vi "OHLayerGen.vi"(6 "Layer":u32=160, 8 "OHL2pow":dbl=150.0, 9 "OHL1pow":dbl=75.0, 10 "HatchPow":T5={"Power"=300.0, "Mark Speed"=400.0, "Jump Speed"=1000.0}, 11 "RectHatch":T6={"Width"=10.0, "Height"=10.0, "Angle"=45.0, "OffX"=0.1, "OffY"=0.1, "Spacing"=0.1} {"Spacing" format="%#_13g"; "OffY" format="%#_13g"; "OffX" format="%#_13g"; "Height" format="%#_13g"; "Width" format="%#_13g"}) -> (3 "PathSups":T1[](array[typedef]))   [LabVIEW 2014]
uses:
  TypeDefs/RectHatch.ctl
  TypeDefs/PowerSpeed.ctl
  TypeDefs/PathSupreme.ctl
  PSup2SCAN/Sub/VelocityProfile.ctl
  PSup2SCAN/Sub/PathCut.ctl
  PSup2SCAN/Sub/Segment.ctl
  PSup2SCAN/Sub/Point.ctl
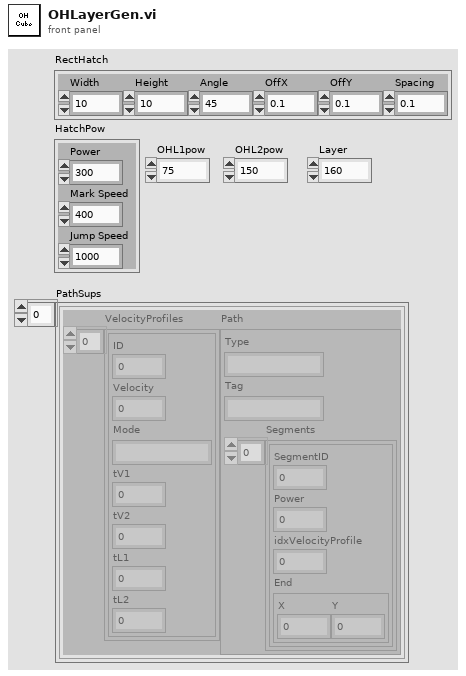
[diagram p1: front panel]
types:
  T1 = typedef "PathSupreme.ctl" = cluster{"VelocityProfiles":T2[], "Path":T3}
  T2 = typedef "VelocityProfile.ctl" = cluster{"ID":u32, "Velocity":dbl, "Mode":string, "tV1":u32, "tV2":u32, "tL1":u32, "tL2":u32}
  T3 = typedef "PathCut.ctl" = cluster{"Type":string, "Tag":string, "Segments":T4[]}
  T4 = typedef "Segment.ctl" = cluster{"SegmentID":u16, "Power":sgl, "idxVelocityProfile":u16, "End":cluster{"X":sgl, "Y":sgl}}
  T5 = typedef "PowerSpeed.ctl" = cluster{"Power":dbl, "Mark Speed":dbl, "Jump Speed":dbl}
  T6 = typedef "RectHatch.ctl" = cluster{"Width":dbl, "Height":dbl, "Angle":sgl, "OffX":dbl, "OffY":dbl, "Spacing":dbl}
  T7 = typedef "Point.ctl" = cluster{"X":dbl, "Y":dbl}
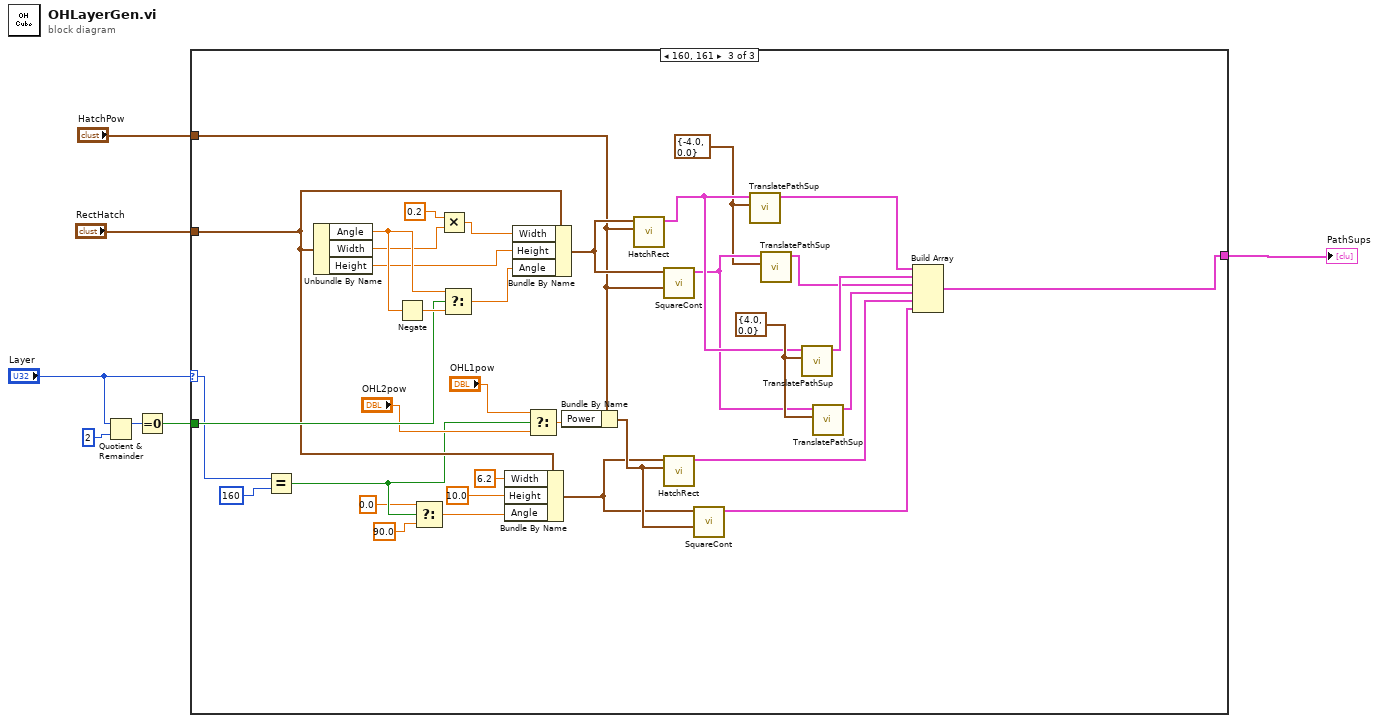
[diagram p0: block diagram]
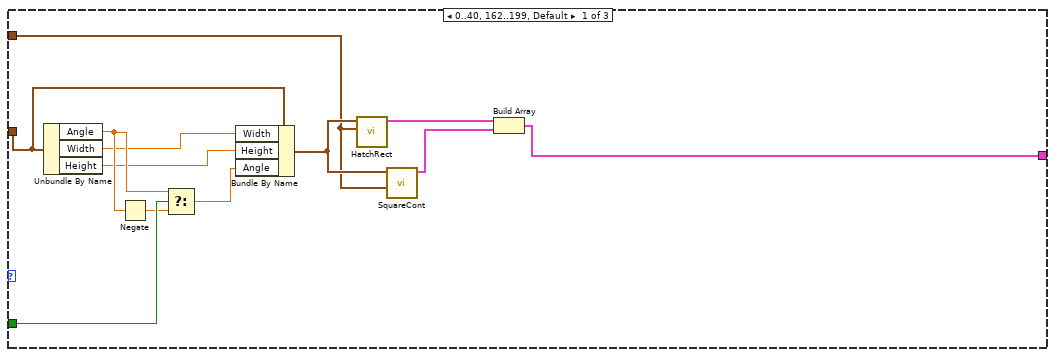
[diagram p2: hidden frame]
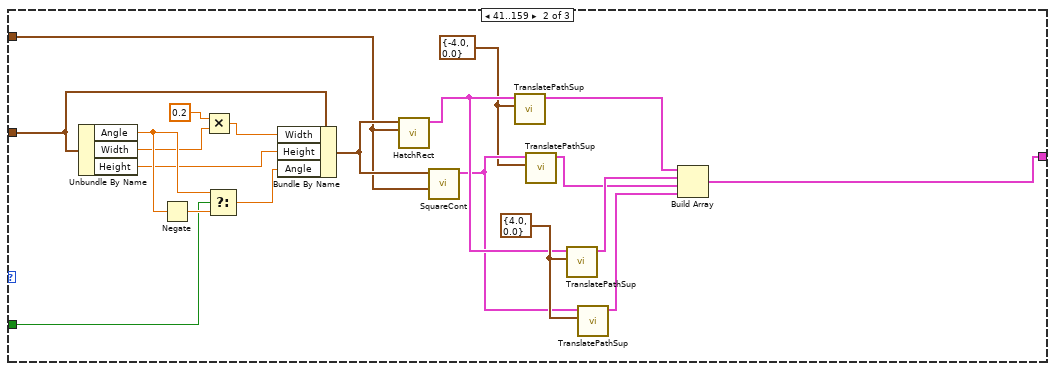
[diagram p3: hidden frame]
diagram:
  n1 = Quotient & Remainder(x="Layer", y=u8 2) -> (x-y*floor(x/y)=w7:u32)  [unwired: 1 out]
  n2 = Equal To 0?(x=w7) -> (x = 0?=w4:bool)
  n3 = case shown="160, 161" "Layer" {
    selector: "Layer" -> [_ _ w48]
    tunnel: w4 -> [w19 w34 w58]
    tunnel: "RectHatch" -> [w18 w33 w55]
    tunnel: "HatchPow" -> [w11 w35 w57]
    tunnel: [w12 w25 w49] -> w1
    frame 0..40, 162..199, Default {
      n4 = Unbundle By Name(w18) -> ("Angle"=w16:sgl, "Width"=w9:dbl, "Height"=w8:dbl)
      n5 = Negate(x=w16) -> (-x=w17:sgl)
      n6 = Select(t=w16, s=w19, f=w17) -> (s? t:f=w15:sgl)
      n7 = Bundle By Name(cluster=w18, "Width"=w9, "Height"=w8, "Angle"=w15) -> (w14:T6)
      n8 = call "HatchRect.vi"("HatchPow"=w11, "RectHatch"=w14) -> ("PathSupreme"=w13:T1)  [unwired: 9 in]
      n9 = call "SquareCont.vi"("ContPow"=w11, "RectHatch"=w14) -> ("PathSupreme"=w10:T1)  [unwired: 9 in]
      n10 = Build Array(w13, w10) -> (w12:T1[])
    }
    frame 41..159 {
      w20 = T7 {"X"=-4.0, "Y"=0.0} ("Offset")
      w32 = T7 {"X"=4.0, "Y"=0.0} ("Offset")
      n11 = Unbundle By Name(w33) -> ("Angle"=w38:sgl, "Width"=w22:dbl, "Height"=w24:dbl)
      n12 = Negate(x=w38) -> (-x=w39:sgl)
      n13 = Multiply(x=0.2 ("Width"), y=w22) -> (x*y=w21:dbl)
      n14 = Select(t=w38, s=w34, f=w39) -> (s? t:f=w37:sgl)
      n15 = Bundle By Name(cluster=w33, "Width"=w21, "Height"=w24, "Angle"=w37) -> (w36:T6)
      n16 = call "HatchRect.vi"("HatchPow"=w35, "RectHatch"=w36) -> ("PathSupreme"=w31:T1)  [unwired: 9 in]
      n17 = call "SquareCont.vi"("ContPow"=w35, "RectHatch"=w36) -> ("PathSupreme"=w30:T1)  [unwired: 9 in]
      n18 = call "TranslatePathSup.vi"("Offset"=w20, "PathSupreme"=w31) -> ("PathSupOut"=w29:T1)  [unwired: 9 in]
      n19 = call "TranslatePathSup.vi"("Offset"=w20, "PathSupreme"=w30) -> ("PathSupOut"=w27:T1)  [unwired: 9 in]
      n20 = call "TranslatePathSup.vi"("Offset"=w32, "PathSupreme"=w31) -> ("PathSupOut"=w28:T1)  [unwired: 9 in]
      n21 = call "TranslatePathSup.vi"("Offset"=w32, "PathSupreme"=w30) -> ("PathSupOut"=w26:T1)  [unwired: 9 in]
      n22 = Build Array(w29, w28, w27, w26) -> (w25:T1[])
    }
    frame 160, 161 {
      w59 = T7 {"X"=-4.0, "Y"=0.0} ("Offset")
      w70 = T7 {"X"=4.0, "Y"=0.0} ("Offset")
      n23 = Equal?(x=w48, y=u32 160) -> (x = y?=w43:bool)
      n24 = Unbundle By Name(w55) -> ("Angle"=w73:sgl, "Width"=w61:dbl, "Height"=w63:dbl)
      n25 = Negate(x=w73) -> (-x=w74:sgl)
      n26 = Select(t=sgl 0.0 ("Angle"), s=w43, f=sgl 90.0 ("Angle")) -> (s? t:f=w40:sgl)
      n27 = Multiply(x=0.2 ("Width"), y=w61) -> (x*y=w60:dbl)
      n28 = Select(t=w73, s=w58, f=w74) -> (s? t:f=w72:sgl)
      n29 = Bundle By Name(cluster=w55, "Width"=6.2, "Height"=10.0, "Angle"=w40) -> (w52:T6)
      n30 = Bundle By Name(cluster=w55, "Width"=w60, "Height"=w63, "Angle"=w72) -> (w71:T6)
      n31 = Select(t="OHL1pow", s=w43, f="OHL2pow") -> (s? t:f=w46:dbl)
      n32 = Bundle By Name(cluster=w57, "Power"=w46) -> (w56:T5)
      n33 = call "HatchRect.vi"("HatchPow"=w57, "RectHatch"=w71) -> ("PathSupreme"=w69:T1)  [unwired: 9 in]
      n34 = call "SquareCont.vi"("ContPow"=w57, "RectHatch"=w71) -> ("PathSupreme"=w68:T1)  [unwired: 9 in]
      n35 = call "HatchRect.vi"("HatchPow"=w56, "RectHatch"=w52) -> ("PathSupreme"=w51:T1)  [unwired: 9 in]
      n36 = call "SquareCont.vi"("ContPow"=w56, "RectHatch"=w52) -> ("PathSupreme"=w50:T1)  [unwired: 9 in]
      n37 = call "TranslatePathSup.vi"("Offset"=w59, "PathSupreme"=w69) -> ("PathSupOut"=w67:T1)  [unwired: 9 in]
      n38 = call "TranslatePathSup.vi"("Offset"=w59, "PathSupreme"=w68) -> ("PathSupOut"=w65:T1)  [unwired: 9 in]
      n39 = call "TranslatePathSup.vi"("Offset"=w70, "PathSupreme"=w69) -> ("PathSupOut"=w66:T1)  [unwired: 9 in]
      n40 = call "TranslatePathSup.vi"("Offset"=w70, "PathSupreme"=w68) -> ("PathSupOut"=w64:T1)  [unwired: 9 in]
      n41 = Build Array(w67, w66, w65, w64, w51, w50) -> (w49:T1[])
    }
  }
  "PathSups" <- w1
